vi "Day 10 - Cathode Ray Tube.vi"() -> ()   [LabVIEW 2020, in "AoC 2022.lvlib"]
uses:
  AoC 2022.lvlib
panel:
  in  "Dark Pixel":string=" "
  in  "Lit Pixel":string="#"
  in  "Puzzle Input":string="addx 15\naddx -11\naddx 6\naddx -3\naddx 5\naddx -1\naddx -8\naddx 13\naddx 4\nnoop\naddx -1\naddx 5\naddx -1\naddx 5\naddx -1\naddx 5\naddx -1\naddx 5\naddx -1\naddx -35\naddx 1\naddx 24\naddx -19\naddx 1\naddx 16\naddx -11\nnoop\nnoop\naddx 21\naddx -15\nnoop\nnoop\naddx -3\naddx 9\naddx 1\naddx -3\naddx 8\naddx 1\naddx 5\nnoop\nnoop\nnoop\nnoop\nnoop\naddx -36\nnoop\naddx 1\naddx 7\nnoop\nnoop\nnoop\naddx 2\naddx 6\nnoop\nnoop\nnoop\nnoop\nnoop\naddx 1\nnoop\nnoop\naddx 7\naddx 1\nnoop\naddx -13\naddx 13\naddx 7\nnoop\naddx 1\naddx -33\nnoop\nnoop\nnoop\naddx 2\nnoop\nnoop\nnoop\naddx 8\nnoop\naddx -1\naddx 2\naddx 1\nnoop\naddx 17\naddx -9\naddx 1\naddx 1\naddx -3\naddx 11\nnoop\nnoop\naddx 1\nnoop\naddx 1\nnoop\nnoop\naddx -13\naddx -19\naddx 1\naddx 3\naddx 26\naddx -30\naddx 12\naddx -1\naddx 3\naddx 1\nnoop\nnoop\nnoop\naddx -9\naddx 18\naddx 1\naddx 2\nnoop\nnoop\naddx 9\nnoop\nnoop\nnoop\naddx -1\naddx 2\naddx -37\naddx 1\naddx 3\nnoop\naddx 15\naddx -21\naddx 22\naddx -6\naddx 1\nnoop\naddx 2\naddx 1\nnoop\naddx -10\nnoop\nnoop\naddx 20\naddx 1\naddx 2\naddx 2\naddx -6\naddx -11\nnoop\nnoop\nnoop"
  out "Puzzle Part-2 Answer":string
  out "Puzzle Answer":string
  # "Press Ctrl+M & Enter the Puzzle Input and run the VI"
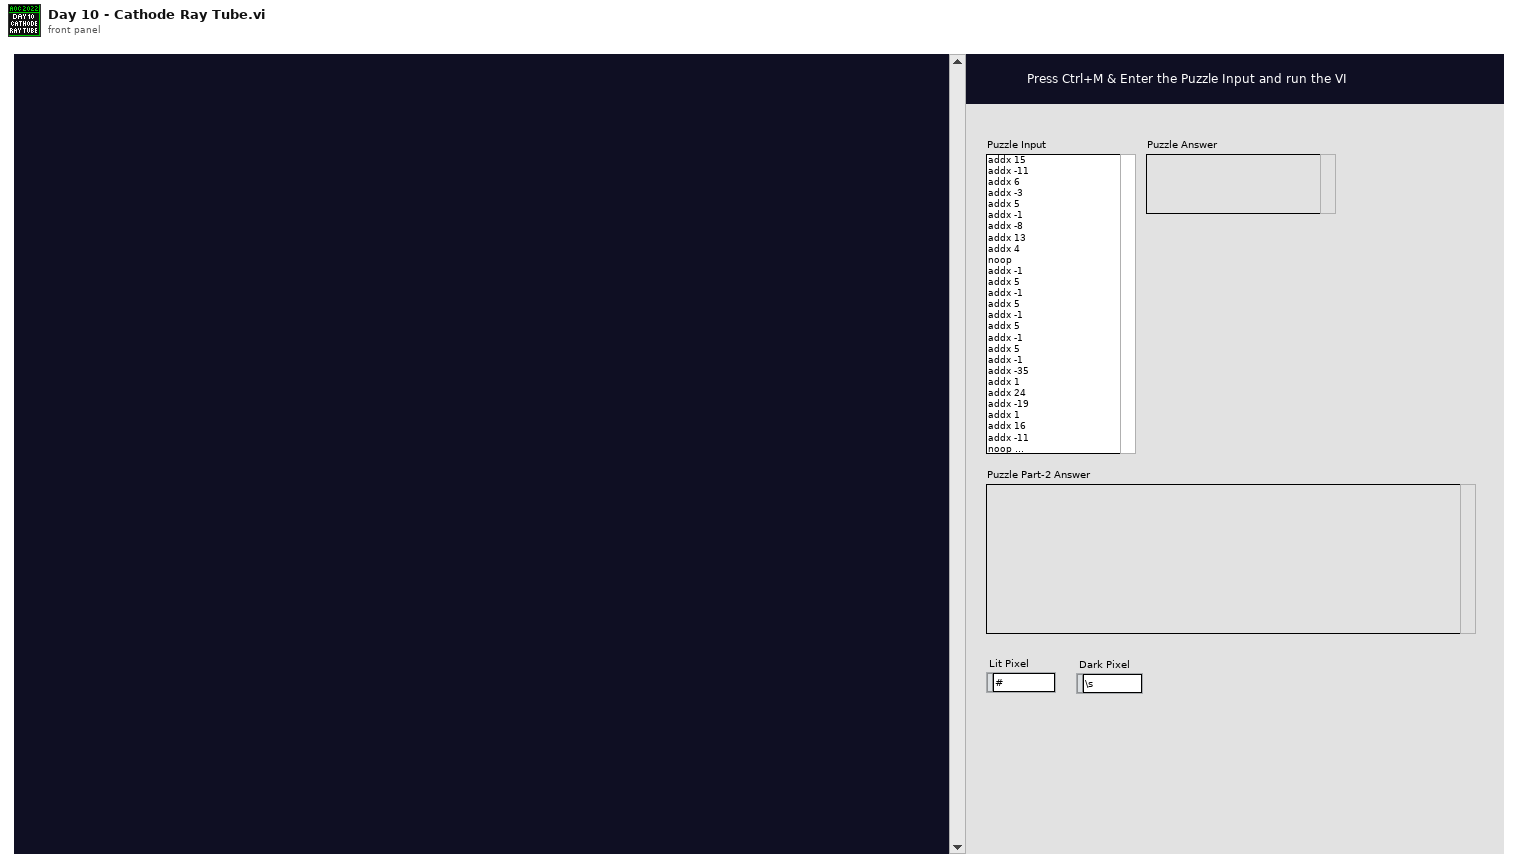
[diagram p1: front panel]
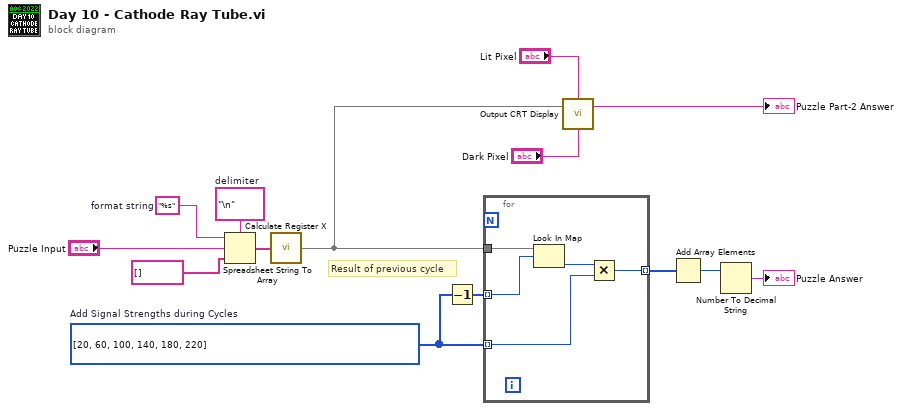
[diagram p0: block diagram]
diagram:
  w2 = i32[] [20, 60, 100, 140, 180, 220]  # Add Signal Strengths during Cycles
  w12 = "%s"  # format string
  w14 = "\n"  # delimiter
  # "Result of previous cycle"
  n1 = Spreadsheet String To Array(delimiter (Tab)=w14, format string=w12, spreadsheet string="Puzzle Input", array type (2D Dbl)=string[] []) -> (array=w10:string[])
  n2 = call "Calculate Register X.vi"("Instructions"=w10) -> ("Register X"=w6:map{i32, i32})
  n3 = Decrement(x=w2) -> (x-1=w1:i32[])
  n4 = for {
    tunnel: w6 -> [w19]
    tunnel: w2 -> [w17] mode=indexing
    tunnel: [w16] -> w7 mode=indexing
    tunnel: w1 -> [w15] mode=indexing
    n5 = Look In Map(map=w19, key=w15) -> (value=w18:i32)  [unwired: 1 in, 1 out]
    n6 = Multiply(x=w18, y=w17) -> (x*y=w16:i32)
  }
  n7 = call "Output CRT Display.vi"("Dark Pixel (.)"="Dark Pixel", "Register X"=w6, "Lit Pixel (#)"="Lit Pixel") -> ("CRT Display"=→"Puzzle Part-2 Answer":string)  [unwired: 2 in]
  n8 = Add Array Elements(numeric array=w7) -> (sum=w9:i32)
  n9 = Number To Decimal String(number=w9) -> (decimal integer string=→"Puzzle Answer":string)  [unwired: 1 in]
